vi "StopTask.vi"(8 "error in (no error)":errorcluster, 11 "NI_DAQmx(AI) in":refnum<class "NI_DAQmx(AI).lvclass">) -> (0 "error out":errorcluster, 3 "NI_DAQmx(AI) out":refnum<class "NI_DAQmx(AI).lvclass">)   [LabVIEW 2025, in "NI_DAQmx(AI).lvclass"]
uses:
  NI_DAQmx(AI).lvclass
  NI_DAQmx(AI).lvclass/NI_DAQmx(AI).ctl
  Read task.vi
  DAQ_Abstr/Task_Type/AI_Task/AI_Task/AI_Task.lvclass
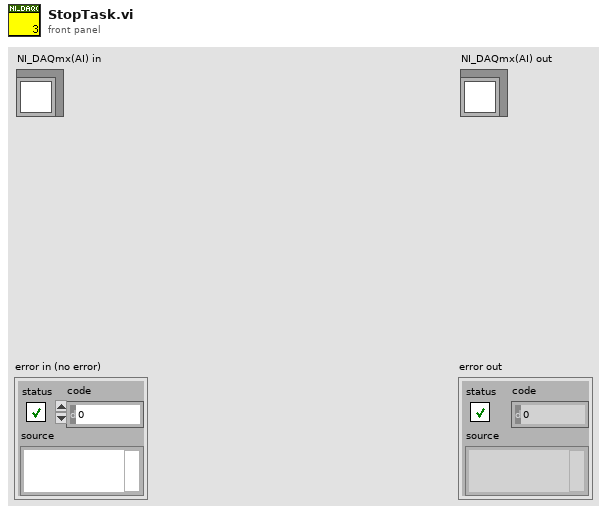
[diagram p1: front panel]
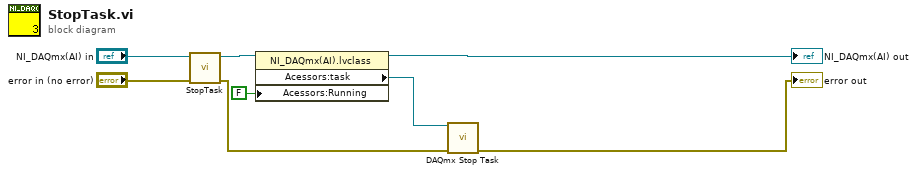
[diagram p0: block diagram]
diagram:
  n1 = call-parent "StopTask.vi"("error in (no error)"="error in (no error)", "Task_Abstr in"="NI_DAQmx(AI) in") -> ("error out"=w3:errorcluster, "Task_Abstr out"=w8:refnum<class "NI_DAQmx(AI).lvclass">)  [unwired: 8 in]
  n2 = property class="NI_DAQmx(AI).lvclass"(reference=w8, "Acessors:Running"=FALSE ("Running")) -> (reference out=→"NI_DAQmx(AI) out":refnum<class "NI_DAQmx(AI).lvclass">, "Acessors:task"=w4:refnum<k21>)  [unwired: 1 in, 1 out]
  n3 = call <vilib>:"DAQmx Stop Task.vi"("task/channels in"=w4, "error in"=w3) -> ("error out"=→"error out":errorcluster)  [unwired: 12 in, 1 out]
